vi "Wait for Generation State.vi"(0 "fpga interface in":refnum<k20>, 5 "state mask":T2[](array[typedef]), 7 "timeout (s)":dbl, 9 "error on timeout":bool=TRUE, 11 "error in (no error)":errorcluster) -> (4 "fpga interface out":refnum<k20>, 6 "state matches":bool, 8 "state":T1(ring), 15 "error out":errorcluster)   [LabVIEW 2023, in "GettingStarted_Gen_148X_Host.lvlib"]
uses:
  GettingStarted_Gen_148X_Host.lvlib
  <instrlib>/FlexRIO/CSI-2/v2/FPGA/Types/Generation Engine State.ctl
  Types/148x_Gen_FPGA_Reference.ctl
  <vilib>/rvi/errors/niLvFpgaAdjustHostInterfaceError.vi
  <vilib>/rvi/interface/nirviReadWriteControl/nirviReadWriteControl.xnode
  NiFpgaLv.dll
  <vilib>/rvi/interface/Simulation/niFpgaSimulationCallBeginRW.vi
  <instrlib>/FlexRIO/CSI-2/v2/FPGA/NI CSI-2 API FPGA v2.lvlib
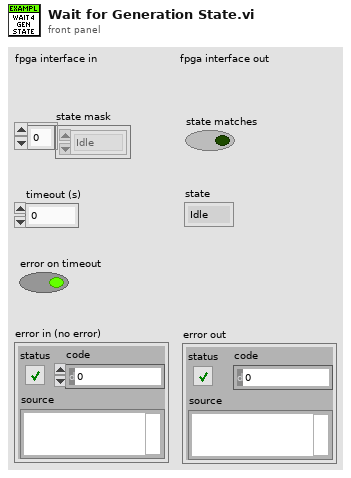
[diagram p1: front panel]
types:
  T1 = enum8{"Idle", "Ready For Start Trigger", "Generate Packets", "Done", "Error"}
  T2 = typedef "NI CSI-2 API FPGA v2.lvlib/Generation Engine State.ctl" = enum8{"Idle", "Ready For Start Trigger", "Generate Packets", "Done", "Error"}
  T3 = typedef "GettingStarted_Gen_148X_Host.lvlib/148x_Gen_FPGA_Reference.ctl" = refnum<k20>
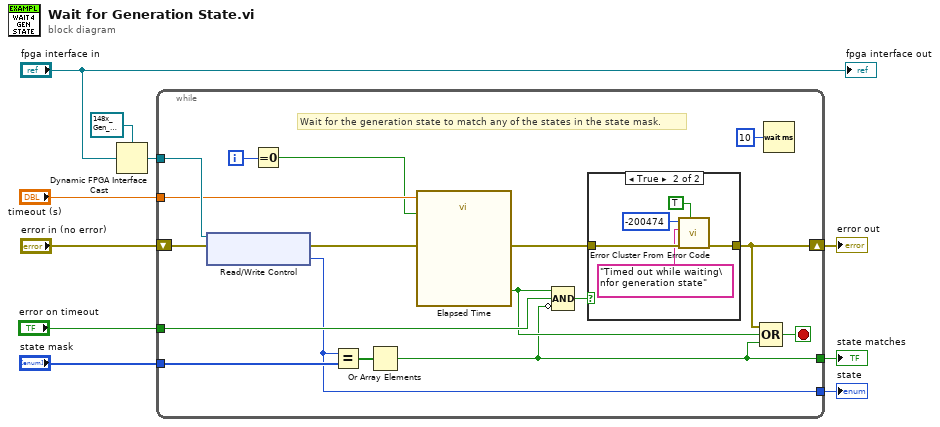
[diagram p0: block diagram]
diagram:
  n1 = Dynamic FPGA Interface Cast(Session In=T3 refnum ("FPGA VI Reference Out"), Type="fpga interface in") -> (Session Out=w4:T3)
  n2 = while {
    tunnel: w4 -> [w27]
    shift-right: [w21] -> w6
    shift-left: "error in (no error)" -> [w25]
    tunnel: "timeout (s)" -> [w23]
    tunnel: "state mask" -> [w17]
    tunnel: "error on timeout" -> [w15]
    tunnel: [w13] -> w10
    tunnel: [w12] -> w1
    i -> [w19]
    stop <- w26 stop-if-true
    # "Wait for the generation state to match any of the states in the state mask."
    n3 = xnode "Read/Write Control"("FPGA VI Reference In"=w27, "error in"=w25) -> ("error out"=w24:errorcluster, "generation state"=w12:T1)  [unwired: 1 out]
    n4 = Equal To 0?(x=w19) -> (x = 0?=w18:bool)
    n5 = Equal?(x=w12, y=w17) -> (x = y?=w16:bool[])
    n6 = Or Array Elements(Boolean array=w16) -> (logical OR=w13:bool)
    n7 = call "Elapsed Time"("Time Target (s)"=w23, "Reset"=w18, "error in (no error)"=w24) -> ("Time has Elapsed"=w14:bool, "error out"=w22:errorcluster)  [unwired: 9 in, 6 out]
    n8 = Compound Arithmetic op=AND(w14, w15, invert w13) -> (w20:bool)
    n9 = case shown="True" w20 {
      tunnel: w22 -> [w28 w32]
      tunnel: [w28 w31] -> w21
      frame False {
      }
      frame True {
        n10 = call <vilib>:"Error Cluster From Error Code.vi"("show call chain? (False)"=TRUE, "error in (no error)"=w32, "error message (\"\")"="Timed out while waiting\nfor generation state" ("error message (\"\")"), "error code (0)"=-200474) -> ("error out"=w31:errorcluster)  [unwired: 5 in]
      }
    }
    n11 = Compound Arithmetic op=OR(w21, w14, w13) -> (w26:bool)
    n12 = Wait (ms)(milliseconds to wait=u32 10) -> ()  [unwired: 1 out]
  }
  "state matches" <- w10
  "error out" <- w6
  "state" <- w1
  "fpga interface out" <- "fpga interface in"
